vi "新剖面数据上传.vi"(11 "错误输入（无错误）":errorcluster) -> (15 "error out":errorcluster)   [LabVIEW 2016, in "数据传输系统-04.lvlib"]
uses:
  <vilib>/Utility/config.llb/Write Key (String).vi
  <vilib>/Utility/config.llb/Read Key (String).vi
  <vilib>/Utility/config.llb/NI_LVConfig.lvlib
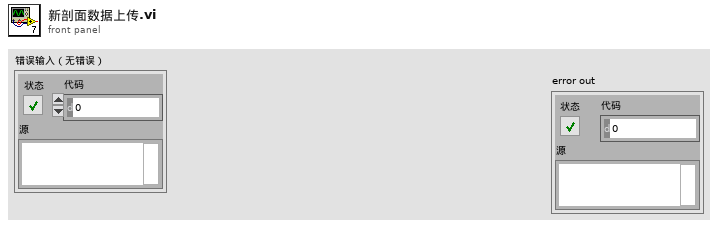
[diagram p1: front panel]
types:
  T1 = cluster{"setini":string, "sysini":string, "hechaini":string, "actualwrite":string, "actualread":string, "datasent":string, "反控命令信息队列":string, "反控与仪器交互":string}
  T2 = typedef "NI_LVConfig.lvlib/Config Data RefNum.ctl" = refnum<k1>
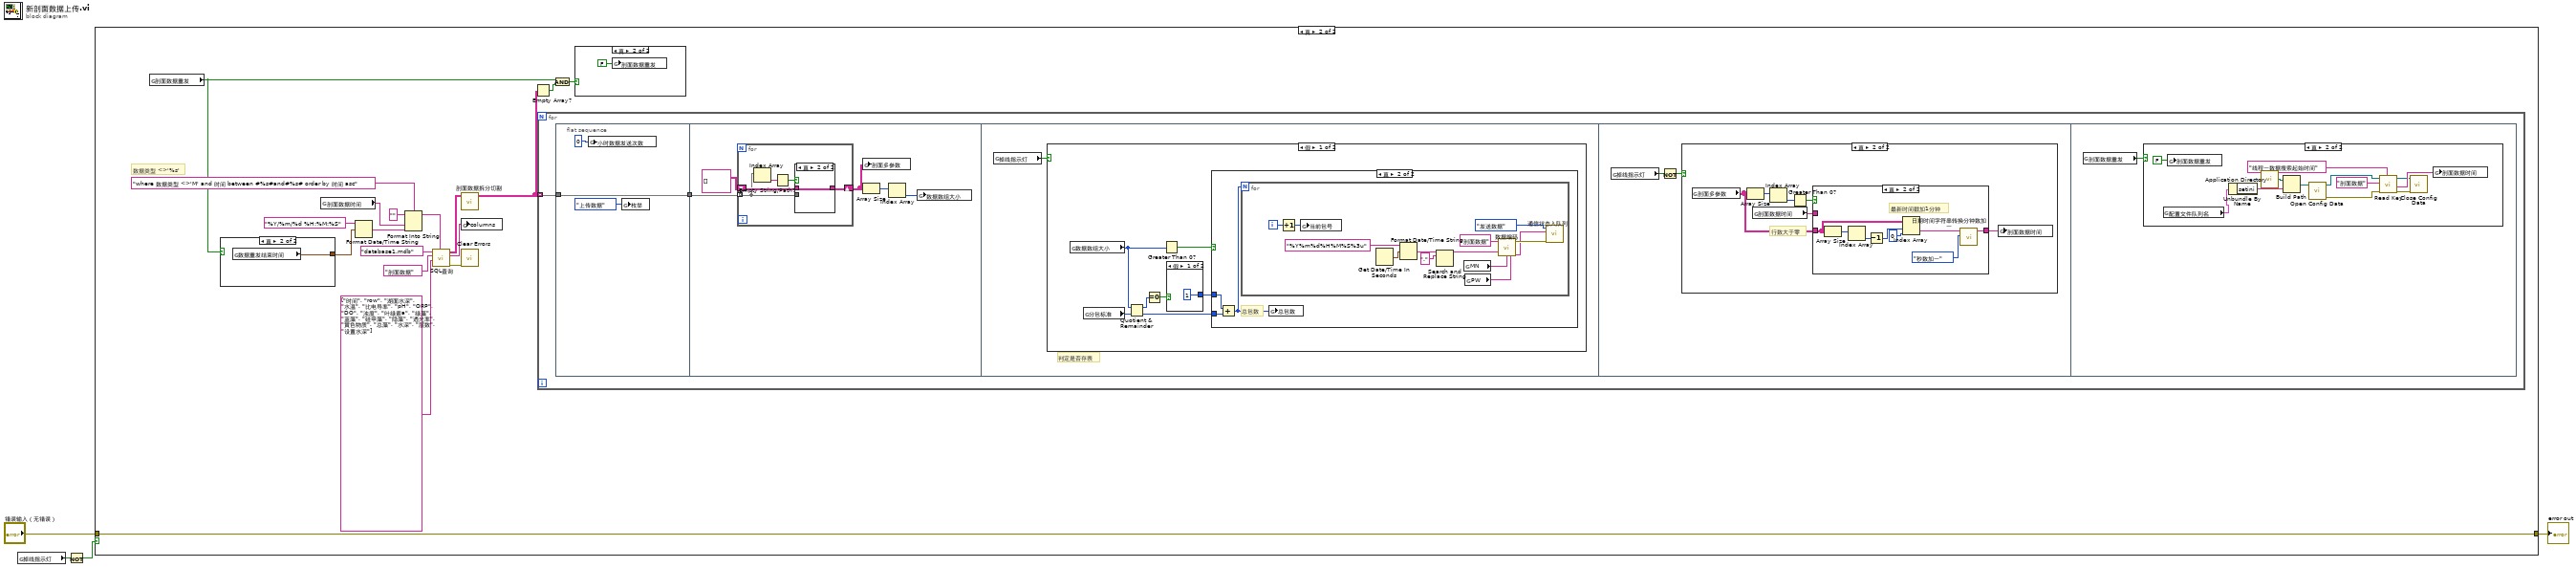
[diagram p0: block diagram]
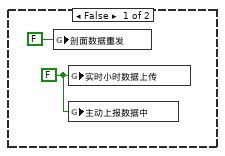
[diagram p2: hidden frame]
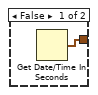
[diagram p4: hidden frame]
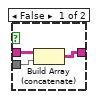
[diagram p5: hidden frame]
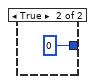
[diagram p6: hidden frame]
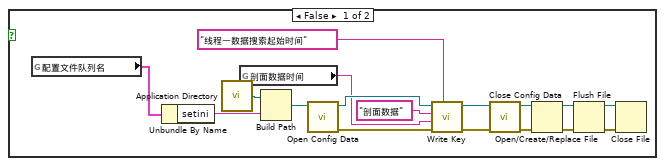
[diagram p11: hidden frame]
diagram:
  n1 = global read "全局 数据发送重叠.vi" "掉线指示灯"() -> (w4:bool)
  n2 = Not(x=w4) -> (.not. x?=w1:bool)
  n3 = case shown="真" w1 {
    tunnel: [_ w24] -> w3
    tunnel: "错误输入（无错误）" -> [_ w24]
    frame False {
      w6 = FALSE ("小时数据上传")
      n4 = global write "断电保存全局.vi" "剖面数据重发"(FALSE ("剖面数据重发")) -> ()
      n5 = global write "全局1.vi" "实时小时数据上传"(w6) -> ()
      n6 = global write "全局 数据发送重叠.vi" "主动上报数据中"(w6) -> ()
    }
    frame True {
      # "数据类型 <>'%s'"
      n7 = global read "断电保存全局.vi" "剖面数据重发"() -> (w7:bool)
      n8 = case shown="真" w7 {
        tunnel: [w26 w27] -> w11
        frame False {
          n9 = Get Date/Time In Seconds() -> (seconds since 1Jan1904=w26:timestamp)
        }
        frame True {
          n10 = global read "断电保存全局.vi" "数据重发结束时间"() -> (w27:timestamp)
        }
      }
      n11 = global read "全局 水样时间.vi" "剖面数据时间"() -> (w17:string)
      n12 = Format Date/Time String(time format string (%c)="%Y/%m/%d %H:%M:%S" ("时间格式字符串(%c)"), seconds (now)=w11) -> (date/time string=w16:string)  [unwired: 1 in]
      n13 = Format Into String(format string="where 数据类型 <>'M' and 时间 between #%s#and#%s# order by 时间 asc" ("condition"), initial string="" ("初始字符串"), w17, w16) -> (resulting string=w15:string)  [unwired: 1 in, 1 out]
      n14 = call "SQL查询.vi"("condition"=w15, "columns"=string[] ["时间", "row", "湖面水深", "水温", "比电导率", "pH", "ORP", "DO", "浊度", "叶绿素a", "绿藻", "蓝藻", "硅甲藻", "隐藻", "透光率", "黄色物质", "总藻", "水深", "层数", "设置水深"], "table输入"="剖面数据", "database"="database1.mdb") -> ("error out"=w13:errorcluster, "columns输出"=w14:string[], "data"=w23:string[][])  [unwired: 4 in, 1 out]
      n15 = call "剖面数据拆分切割.vi"("剖面多参数输入"=w23) -> ("剖面多参数输出"=w10:string[][][])  [unwired: 10 in]
      n16 = global write "全局 所有参数.vi" "columns"(w14) -> ()
      n17 = call <vilib>:"Clear Errors.vi"("error in (no error)"=w13) -> ()  [unwired: 5 in, 2 out]
      n18 = Empty Array?(array=w10) -> (empty?=w9:bool)
      n19 = for {
        tunnel: w10 -> [w29] mode=indexing
        n20 = flat-sequence {
          tunnel: w29 -> [w32]
          tunnel: [w32] -> w28
          tunnel: w28 -> [w35]
          frame #0 {
            n21 = global write "全局 小时数据发送次数.vi" "小时数据发送次数"(0 ("小时数据发送次数")) -> ()
            n22 = global write "全局1.vi" "枚举"(enum16{"返回请求应答", "上传数据", "返回执行结果"}."上传数据" ("枚举")) -> ()
          }
          frame #1 {
            n23 = for {
              tunnel: w35 -> [w40] mode=indexing
              shift-right: [w41] -> w33
              shift-left: string[][] [] ("剖面多参数输入") -> [w42]
              n24 = Index Array(array=w40) -> (element=w39:string)  [unwired: 1 in]
              n25 = Empty String/Path?(string/path=w39) -> (empty?=w38:bool)
              n26 = case shown="真" w38 {
                tunnel: w42 -> [w45 w46]
                tunnel: w40 -> [w44 _]
                tunnel: [w43 w46] -> w41
                frame False {
                  n27 = Build Array (concatenate)(w45, w44) -> (w43:string[][])
                }
                frame True {
                }
              }
            }
            n28 = global write "全局 所有参数.vi" "剖面多参数"(w33) -> ()
            n29 = Array Size(array=w33) -> (size(s)=w36:i32[])
            n30 = Index Array(array=w36) -> (element=w37:i32)  [unwired: 1 in]
            n31 = global write "全局 数据数组大小.vi" "数据数组大小"(w37) -> ()
          }
          frame #2 {
            # "判定是否存表"
            n32 = global read "全局 数据发送重叠.vi" "掉线指示灯"() -> (w47:bool)
            n33 = case shown="假" w47 {
              frame False {
                n34 = global read "全局 数据数组大小.vi" "数据数组大小"() -> (w53:i32)
                n35 = global read "全局 数据数组大小.vi" "分包标准"() -> (w51:i32)
                n36 = Quotient & Remainder(x=w53, y=w51) -> (x-y*floor(x/y)=w50:i32, floor(x/y)=w52:i32)
                n37 = Equal To 0?(x=w50) -> (x = 0?=w49:bool)
                n38 = Greater Than 0?(x=w53) -> (x > 0?=w54:bool)
                n39 = case shown="假" w49 {
                  tunnel: [1 ("x") 0 ("x")] -> w48
                  frame False {
                  }
                  frame True {
                  }
                }
                n40 = case shown="真" w54 {
                  tunnel: w52 -> [_ w59]
                  tunnel: w48 -> [_ w57]
                  frame False {
                  }
                  frame True {
                    # "总包数"
                    n41 = Add(x=w57, y=w59) -> (x+y=w58:i32)
                    n42 = for {
                      N: w58 -> [_]
                      i -> [w64]
                      n43 = Increment(x=w64) -> (x+1=w63:i32)
                      n44 = global write "全局 数据数组大小.vi" "当前包号"(w63) -> ()
                      n45 = Get Date/Time In Seconds() -> (seconds since 1Jan1904=w70:timestamp)
                      n46 = Format Date/Time String(time format string (%c)="%Y%m%d%H%M%S%3u" ("时间格式字符串(%c)"), seconds (now)=w70) -> (date/time string=w69:string)  [unwired: 1 in]
                      n47 = Search and Replace String(input string=w69, search string="." ("搜索字符串")) -> (result string=w67:string)  [unwired: 6 in, 3 out]
                      n48 = global read "断电保存全局.vi" "MN"() -> (w60:string)
                      n49 = global read "断电保存全局.vi" "PW"() -> (w66:string)
                      n50 = call "数据编码.vi"("table输入"="剖面数据" ("新元素/子数组"), "QN"=w67, "MN"=w60, "PW"=w66) -> ("错误常量"=w65:errorcluster, "通讯包字符串"=w61:string)  [unwired: 10 in]
                      n51 = call "通信状态入队列.vi"("错误输入（无错误）"=w65, "发送报文"=w61, "枚举"=enum16{"打开连接", "发送数据", "读取数据", "数据处理", "关闭连接"}."发送数据") -> ()  [unwired: 8 in, 1 out]
                    }
                    n52 = global write "全局 数据数组大小.vi" "总包数"(w58) -> ()
                  }
                }
              }
              frame True {
              }
            }
          }
          frame #3 {
            n53 = global read "全局 数据发送重叠.vi" "掉线指示灯"() -> (w73:bool)
            n54 = Not(x=w73) -> (.not. x?=w74:bool)
            n55 = case shown="真" w74 {
              frame False {
              }
              frame True {
                # "行数大于零"
                n56 = global read "全局 所有参数.vi" "剖面多参数"() -> (w79:string[][])
                n57 = Array Size(array=w79) -> (size(s)=w76:i32[])
                n58 = global read "全局 水样时间.vi" "剖面数据时间"() -> (w80:string)
                n59 = Index Array(array=w76) -> (element=w77:i32)  [unwired: 1 in]
                n60 = Greater Than 0?(x=w77) -> (x > 0?=w78:bool)
                n61 = case shown="真" w78 {
                  tunnel: w79 -> [_ w86]
                  tunnel: [w81 w83] -> w75
                  tunnel: w80 -> [w81 _]
                  frame False {
                  }
                  frame True {
                    # "最新时间戳加1分钟"
                    n62 = Array Size(array=w86) -> (size(s)=w88:i32[])
                    n63 = Index Array(array=w88) -> (element=w87:i32)  [unwired: 1 in]
                    n64 = Decrement(x=w87) -> (x-1=w85:i32)
                    n65 = Index Array(array=w86, index (row)=w85, index (col)=0 ("禁用的索引 (列)")) -> (element=w89:string)
                    n66 = call "日期时间字符串转换分钟数加一.vi"("枚举"=enum16{"分钟数加一", "秒数加一", "小时数加一"}."秒数加一", "data[0]"=w89) -> ("日期/时间字符串"=w83:string)  [unwired: 9 in]
                  }
                }
                n67 = global write "全局 水样时间.vi" "剖面数据时间"(w75) -> ()
              }
            }
          }
          frame #4 {
            n68 = global read "断电保存全局.vi" "剖面数据重发"() -> (w90:bool)
            n69 = case shown="真" w90 {
              frame False {
                n70 = global read "全局1.vi" "配置文件队列名"() -> (w91:T1)
                n71 = Unbundle By Name(w91) -> ("setini"=w92:string)
                n72 = call <vilib>:"Application Directory.vi"() -> ("Application Directory"=w101:path)
                n73 = global read "全局 水样时间.vi" "剖面数据时间"() -> (w93:string)
                n74 = Build Path(base path=w101, name or relative path=w92) -> (appended path=w102:path)
                n75 = call <vilib>:"Open Config Data.vi"("configuration file path"=w102) -> ("error out"=w104:errorcluster, "refnum"=w103:T2)  [unwired: 8 in, 1 out]
                n76 = call-poly <vilib>:"Write Key.vi"("section"="线程一数据搜索起始时间", "error in (no error)"=w104, "value"=w93, "key"="剖面数据", "refnum"=w103) -> ("error out"=w106:errorcluster, "refnum out"=w105:T2)  [unwired: 4 in, 1 out]
                n77 = call <vilib>:"Close Config Data.vi"("error in (no error)"=w106, "refnum"=w105) -> ("error out"=w94:errorcluster, "file path"=w95:path)  [unwired: 8 in]
                n78 = Open/Create/Replace File(file path (use dialog)=w95, error in=w94) -> (refnum out=w97:refnum<file>, error out=w96:errorcluster)  [unwired: 4 in, 1 out]
                n79 = Flush File(refnum=w97, error in=w96) -> (refnum out=w98:refnum<file>, error out=w99:errorcluster)
                n80 = Close File(refnum=w98, error in=w99) -> ()  [unwired: 2 out]
              }
              frame True {
                n81 = global read "全局1.vi" "配置文件队列名"() -> (w108:T1)
                n82 = global write "断电保存全局.vi" "剖面数据重发"(FALSE ("剖面数据重发")) -> ()
                n83 = Unbundle By Name(w108) -> ("setini"=w116:string)
                n84 = call <vilib>:"Application Directory.vi"() -> ("Application Directory"=w115:path)
                n85 = Build Path(base path=w115, name or relative path=w116) -> (appended path=w117:path)
                n86 = call <vilib>:"Open Config Data.vi"("configuration file path"=w117) -> ("error out"=w112:errorcluster, "refnum"=w111:T2)  [unwired: 8 in, 1 out]
                n87 = call-poly <vilib>:"Read Key.vi"("section"="线程一数据搜索起始时间", "error in (no error)"=w112, "key"="剖面数据", "refnum"=w111) -> ("error out"=w114:errorcluster, "value"=w119:string, "refnum out"=w113:T2)  [unwired: 4 in, 1 out]
                n88 = call <vilib>:"Close Config Data.vi"("error in (no error)"=w114, "refnum"=w113) -> ()  [unwired: 8 in, 2 out]
                n89 = global write "全局 水样时间.vi" "剖面数据时间"(w119) -> ()
              }
            }
          }
        }
      }
      n90 = And(x=w7, y=w9) -> (x .and. y?=w8:bool)
      n91 = case shown="真" w8 {
        frame False {
        }
        frame True {
          n92 = global write "断电保存全局.vi" "剖面数据重发"(FALSE ("剖面数据重发")) -> ()
        }
      }
    }
  }
  "error out" <- w3
